vi "GetPosition.vi"(8 "error in (no error)":errorcluster, 10 "includeWraps":bool=TRUE, 11 "Axis in":refnum<class "Axis.lvclass">) -> (0 "error out":errorcluster, 1 "Velocity":dbl, 2 "scaledPosn":i64, 3 "Axis out":refnum<class "Axis.lvclass">, 4 "Torque":dbl)   [LabVIEW 2020, in "Axis.lvclass"]
uses:
  Axis.lvclass
  Axis.lvclass/Axis.ctl
  C:/Users/Jonathan/Documents/Clearpath SDK/CSharp Examples/CLRWrapper/x64/Debug/CLRWrapper.dll
  CSharp Examples/CLRWrapper/x64/Debug/CLRWrapper.dll
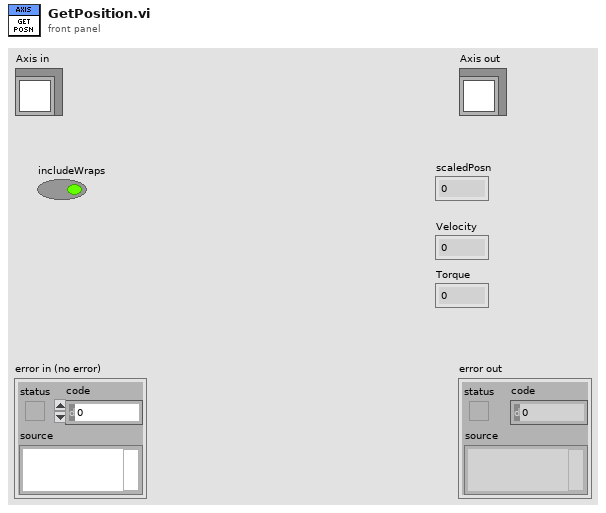
[diagram p1: front panel]
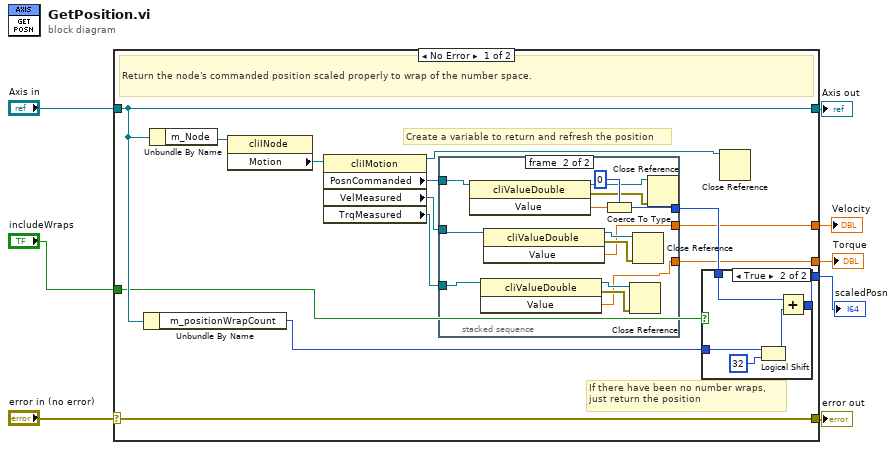
[diagram p0: block diagram]
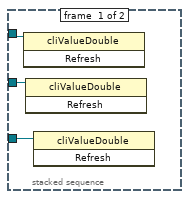
[diagram p3: hidden frame]
diagram:
  n1 = case shown="No Error" "error in (no error)" {
    selector: "error in (no error)" -> [w22 w47]
    tunnel: [w22 w47] -> w7
    tunnel: [w18 w46] -> w5
    tunnel: "Axis in" -> [w18 w46]
    tunnel: "includeWraps" -> [w14 _]
    tunnel: [w16 _] -> w3
    tunnel: [w11 _] -> w2
    tunnel: [w9 _] -> w1
    frame No Error {
      # "Create a variable to return and refresh the position"
      # "If there have been no number wraps, \njust return the position"
      # "Return the node's commanded position scaled properly to wrap of the number space."
      n2 = Unbundle By Name(w18) -> ("m_positionWrapCount"=w15:i64)
      n3 = Unbundle By Name(w18) -> ("m_Node"=w21:refnum<k24>)
      n4 = property class="cliINode"(reference=w21) -> ("Motion"=w20:refnum<k24>)  [unwired: 1 in, 2 out]
      n5 = property class="cliIMotion"(reference=w20) -> (reference out=w13:refnum<k24>, "PosnCommanded"=w19:refnum<k24>, "VelMeasured"=w12:refnum<k24>, "TrqMeasured"=w10:refnum<k24>)  [unwired: 1 in, 1 out]
      n6 = stacked-sequence {
        tunnel: w19 -> [w31 w45]
        tunnel: [_ w43] -> w17
        tunnel: w12 -> [w30 w39]
        tunnel: [_ w36] -> w11
        tunnel: w10 -> [w29 w33]
        tunnel: [_ w32] -> w9
        frame #0 {
          n7 = invoke class="cliValueDouble" method="Refresh"(reference=w31) -> ()  [unwired: 2 in, 3 out]
          n8 = invoke class="cliValueDouble" method="Refresh"(reference=w30) -> ()  [unwired: 2 in, 3 out]
          n9 = invoke class="cliValueDouble" method="Refresh"(reference=w29) -> ()  [unwired: 2 in, 3 out]
        }
        frame #1 {
          n10 = invoke class="cliValueDouble" method="Value"(reference=w45) -> (reference out=w41:refnum<k24>, error out=w40:errorcluster, "Value"=w42:dbl)  [unwired: 2 in]
          n11 = invoke class="cliValueDouble" method="Value"(reference=w33) -> (reference out=w34:refnum<k24>, error out=w35:errorcluster, "Value"=w32:dbl)  [unwired: 2 in]
          n12 = invoke class="cliValueDouble" method="Value"(reference=w39) -> (reference out=w38:refnum<k24>, error out=w37:errorcluster, "Value"=w36:dbl)  [unwired: 2 in]
          n13 = Coerce To Type(0:w42, 1:i64 0) -> (2:w43:i64)
          n14 = Close Reference(reference=w34, error in (no error)=w35) -> ()  [unwired: 1 out]
          n15 = Close Reference(reference=w38, error in (no error)=w37) -> ()  [unwired: 1 out]
          n16 = Close Reference(reference=w41, error in (no error)=w40) -> ()  [unwired: 1 out]
        }
      }
      n17 = case shown="True" w14 {
        tunnel: w17 -> [w23 w24]
        tunnel: [w23 w27] -> w16
        tunnel: w15 -> [_ w26]
        frame False {
        }
        frame True {
          n18 = Logical Shift(y=w26, x=i64 32) -> (x << y=w25:i64)
          n19 = Add(x=w24, y=w25) -> (x+y=w27:i64)
        }
      }
      n20 = Close Reference(reference=w13) -> ()  [unwired: 1 in, 1 out]
    }
    frame Error {
    }
  }
  "error out" <- w7
  "Axis out" <- w5
  "scaledPosn" <- w3
  "Velocity" <- w2
  "Torque" <- w1
